vi "Adv_Register_for_Callback.vi"(8 "error in (no error)":errorcluster, 11 "LightField Automation in":refnum<class "LightField Automation.lvclass">) -> (0 "error out":errorcluster, 3 "LightField Automation out":refnum<class "LightField Automation.lvclass">)   [LabVIEW 2013, in "LightField Automation.lvclass"]
uses:
  LightField Automation.lvclass
  LightField Automation.lvclass/LightField Automation.ctl
  C:/Program Files/Princeton Instruments/LightField/AddInViews/PrincetonInstruments.LightFieldViewV3.dll
  Program Files/Princeton Instruments/LightField/AddInViews/PrincetonInstruments.LightFieldViewV3.dll
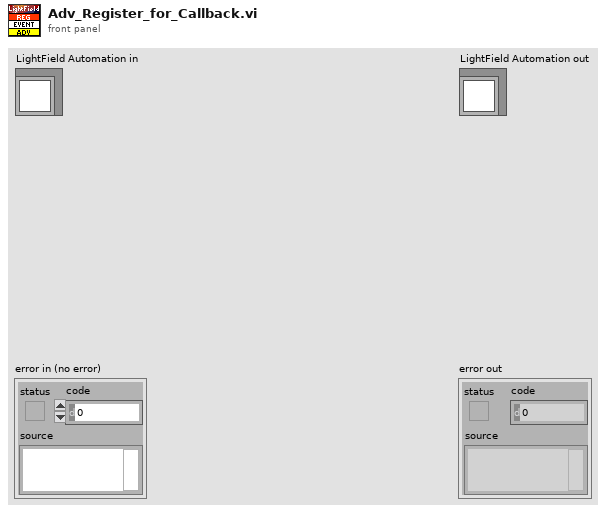
[diagram p1: front panel]
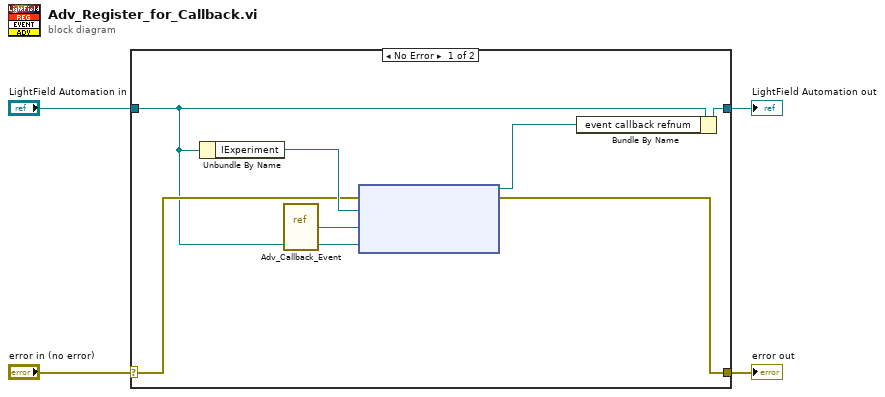
[diagram p0: block diagram]
diagram:
  n1 = case shown="No Error" "error in (no error)" {
    selector: "error in (no error)" -> [w10 w13]
    tunnel: [w9 w13] -> w3
    tunnel: [w8 w12] -> w1
    tunnel: "LightField Automation in" -> [w5 w12]
    frame No Error {
      n2 = Unbundle By Name(w5) -> ("IExperiment"=w11:refnum<k24>)
      n3 = vi-ref "Adv_Callback_Event.vi"() -> ("vi reference"=w6:refnum<vi>)
      n4 = node(w10, w11, w6, w5) -> (w7:refnum<k27>, w9:errorcluster)  [unwired: 1 in]
      n5 = Bundle By Name(cluster=w5, "event callback refnum"=w7) -> (w8:refnum<class "LightField Automation.lvclass">)
    }
    frame Error {
    }
  }
  "error out" <- w3
  "LightField Automation out" <- w1
